vi "GTH_V2.Record2DACPara.vi"(9 "AMP":u8=1 min=1 max=100 step=1, 10 "FREQ":u16, 11 "ParaList":dbl[](array[numeric]) caption="Para List") -> (1 "AMP OUT":u8=1 min=1 max=100 step=1)   [LabVIEW 2012]
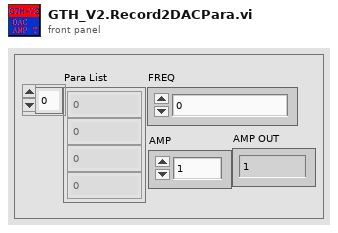
[diagram p1: front panel]
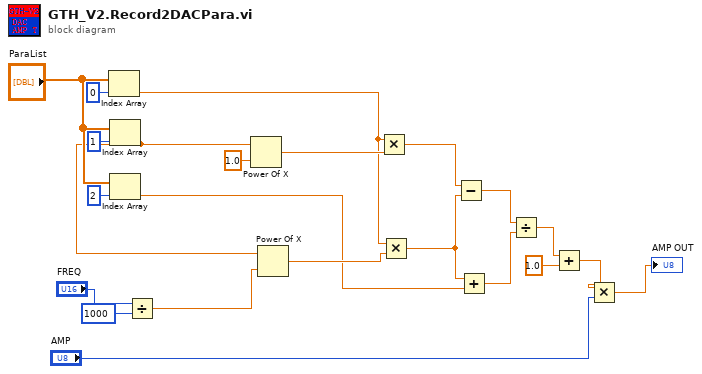
[diagram p0: block diagram]
diagram:
  n1 = Index Array(array="ParaList", index=0 ("索引")) -> (element=w11:dbl)
  n2 = Index Array(array="ParaList", index=1 ("索引")) -> (element=w15:dbl)
  n3 = Index Array(array="ParaList", index=2 ("索引")) -> (element=w7:dbl)
  n4 = Divide(x="FREQ", y=u16 1000) -> (x/y=w13:dbl)
  n5 = Power Of X(1:1.0 ("x"), 2:w15) -> (0:w22:dbl)
  n6 = Power Of X(1:w13, 2:w15) -> (0:w12:dbl)
  n7 = Multiply(x=w11, y=w22) -> (x*y=w10:dbl)
  n8 = Multiply(x=w11, y=w12) -> (x*y=w8:dbl)
  n9 = Subtract(x=w10, y=w8) -> (x-y=w9:dbl)
  n10 = Add(x=w8, y=w7) -> (x+y=w6:dbl)
  n11 = Divide(x=w9, y=w6) -> (x/y=w5:dbl)
  n12 = Add(x=w5, y=1.0) -> (x+y=w3:dbl)
  n13 = Multiply(x=w3, y="AMP") -> (x*y=→"AMP OUT":dbl)
